vi "IS30%_P.vi"() -> ()   [LabVIEW 2020]
panel:
  out "VG IS30% ?":bool
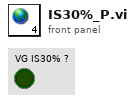
[diagram p1: front panel]
diagram:
